vi "GetText.vi"(8 "error in":errorcluster, 11 "HiPOT Instrument":refnum<class "HiPOT Instrument.lvclass">) -> (0 "error out":errorcluster, 1 "additional text":string, 2 "text":string, 3 "HiPOT Instrument out":refnum<class "HiPOT Instrument.lvclass">, 4 "glyph":string)   [LabVIEW 2025, in "HiPOT.lvlib" / "HiPOT Instrument.lvclass"]
doc: "Copyright 2017 National Instruments Corporation\n\nLicensed under the Apache License, Version 2.0 (the \"License\"); you may not use this file except in compliance with the License. You may obtain a copy of the License at http://www.apache.org/licenses/LICENSE-2.0\nUnless required by applicable law or agreed to in writing, software distributed under the License is distributed on an \"AS IS\" BASIS, WITHOUT WARRANTIES OR CONDITIONS OF ANY KIND, either express or implied. See the License for the specific language governing permissions and limitations under the License."
uses:
  HiPOT Instrument.lvclass
  HiPOT Instrument.lvclass/HiPOT Instrument.ctl
  HiPOT configuration/HiPOT configuration.lvclass
  C:/Users/Public/Documents/Sandia National Labs/TSS Plugin/Abstract Engine.lvlibp/Plugin/Abstract/Instrument configuration/Instrument configuration.lvclass
  Users/Public/Documents/Sandia National Labs/TSS Plugin/Abstract Engine.lvlibp/Plugin/Abstract/Instrument configuration/Read Instrument Setting.vi
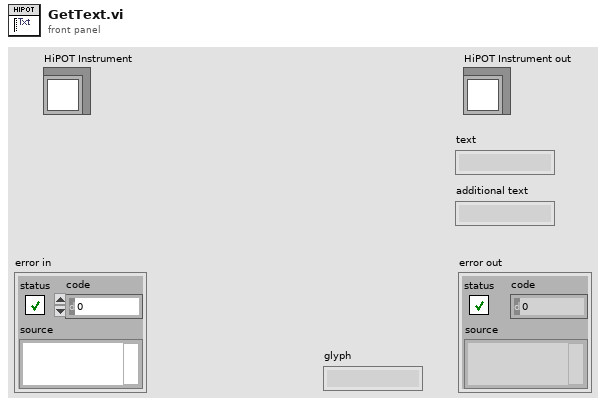
[diagram p1: front panel]
types:
  T1 = cluster{"Type":string, "Engine IP Address":string, "Engine Port":u32, "Address":string, "SW Alias":string, "Description":string, "Enabled":bool, "Model":string, "Serial Number":string, "Asset Number":string, "Calibration Date":string}
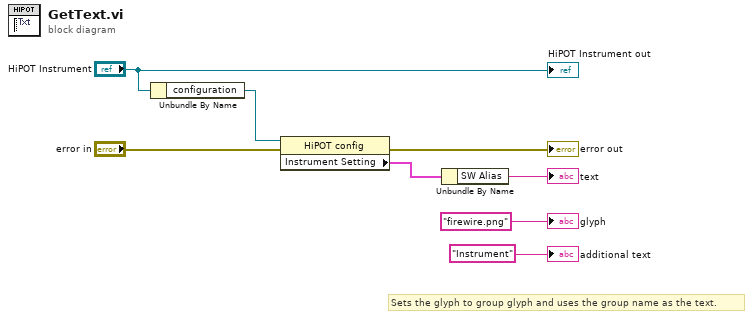
[diagram p0: block diagram]
diagram:
  # "Sets the glyph to group glyph and uses the group name as the text."
  n1 = Unbundle By Name("HiPOT Instrument") -> ("configuration"=w5:refnum<class "HiPOT configuration.lvclass">)
  n2 = property class="HiPOT config"(reference=w5, error in="error in") -> (error out=→"error out":errorcluster, "Instrument Setting"=w1:T1)  [unwired: 1 out]
  n3 = Unbundle By Name(w1) -> ("SW Alias"=→"text":string)
  "additional text" <- "Instrument" ("additional text")
  "glyph" <- "firewire.png" ("glyph")
  "HiPOT Instrument out" <- "HiPOT Instrument"
